vi "Dequeue.vi"(6 "timeout in ms (-1)":i32=-1, 8 "error in (no error)":errorcluster, 11 "Message Queue":T1) -> (0 "error out":errorcluster, 1 "Message Data":variant, 2 "State":T2=enum."Initialize", 3 "Message Queue dub":T1, 4 "timed out?":bool, 5 "Call Chain":string[](array[string]))   [LabVIEW 2019, in "Task Manager.lvlib"]
doc: "This VI pulls messages off the Message Queue."
uses:
  Task Manager.lvlib
  State Name.ctl
  Shared/TypeDefs/Message Queue Ref.ctl
  85968e22-cec5-4834-9408-c5f0918d029d.vi
  0e969a01-278a-410f-94a4-bde872eff04a.vi
  <vilib>/Utility/error.llb/Clear Errors.vi
  <vilib>/Utility/error.llb/Error Cluster From Error Code.vi
panel:
  out "# elements in queue":i32
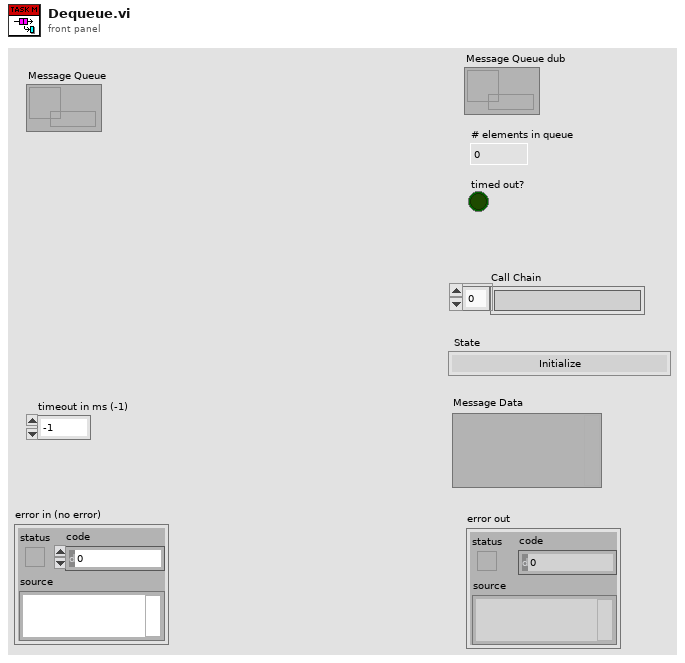
[diagram p1: front panel]
types:
  T1 = typedef "Message Queue Ref.ctl" = refnum<queue>
  T2 = typedef "Task Manager.lvlib/State Name.ctl" = enum16{"Default", "Initialize", "Re-Initialize", "Initialize Data", "Initialize Panel", "[Event Structure] Update Data", "Get Modules", "Add State Info Clone", "Get Queue Sizes", "Get States Calling Info", "Error", "Exit"}
  T3 = cluster{"Custom State Name":string, "Defined State Name":variant, "Call Chain":string[], "Message Data":variant}
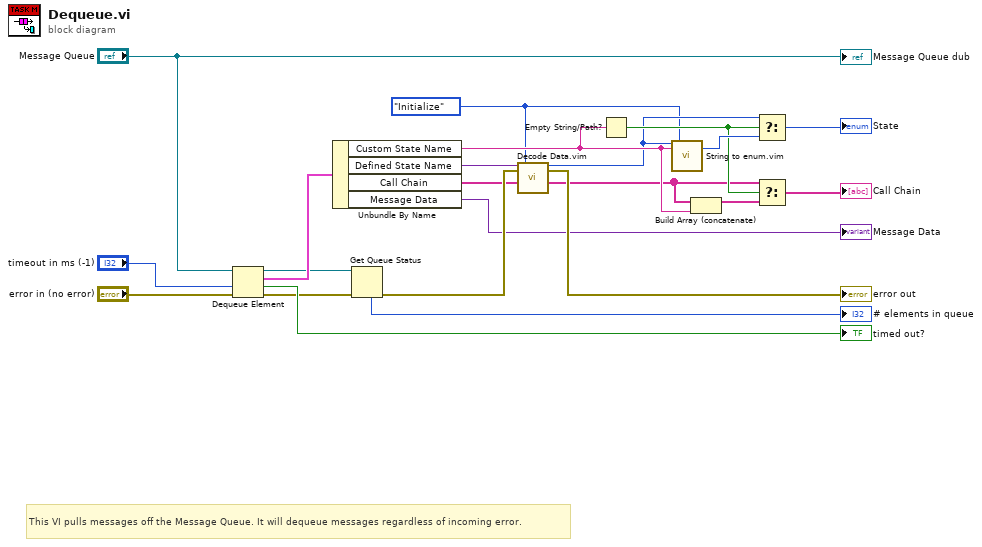
[diagram p0: block diagram]
diagram:
  w1 = State_Name."Initialize" ("State")
  # "This VI pulls messages off the Message Queue. It will dequeue messages regardless of incoming error."
  n1 = Dequeue Element(queue="Message Queue", timeout in ms (-1)="timeout in ms (-1)", error in (no error)="error in (no error)") -> (queue out=w19:T1, element=w21:T3, timed out?=→"timed out?":bool, error out=w16:errorcluster)
  n2 = Unbundle By Name(w21) -> ("Custom State Name"=w6:string, "Defined State Name"=w13:variant, "Call Chain"=w5:string[], "Message Data"=→"Message Data":variant)
  n3 = Get Queue Status(queue=w19, error in (no error)=w16) -> (error out=w12:errorcluster, # elements in queue=→"# elements in queue":i32)  [unwired: 1 in, 6 out]
  n4 = call "Decode Data.vim"("Data"=w13, "error in"=w12, "Type/Default value"=w1) -> ("Data out"=w4:T2, "error out"=→"error out":errorcluster)  [unwired: 15 in]
  n5 = Empty String/Path?(string/path=w6) -> (empty?=w8:bool)
  n6 = call "String to enum.vim"("Enum"=w4, "Item Name"=w6, "Default Item Name"=w1) -> ("Enum Selected"=w9:T2)  [unwired: 14 in, 2 out]
  n7 = Build Array (concatenate)(w5, w6) -> (w7:string[])
  n8 = Select(t=w4, s=w8, f=w9) -> (s? t:f=→"State":T2)
  n9 = Select(t=w5, s=w8, f=w7) -> (s? t:f=→"Call Chain":string[])
  "Message Queue dub" <- "Message Queue"
